vi "DLIbufferedRead.vi"(9 "timeout(ms)":i32, 10 "Ch.":i32, 11 "URL":string) -> (0 "error out":errorcluster, 1 "state(1or0)":i16, 2 "body":string, 3 "headers":string)   [LabVIEW 2016]
uses:
  DLIbufferState.ctl
  ADAM Client/Sub VIs/ADAM Controls/Remember_value_mode.ctl
  <vilib>/httpClient/LabVIEWHTTPClient.lvlib
panel:
  out "allChs":u32 format="%08b"
  out "age(s)":dbl
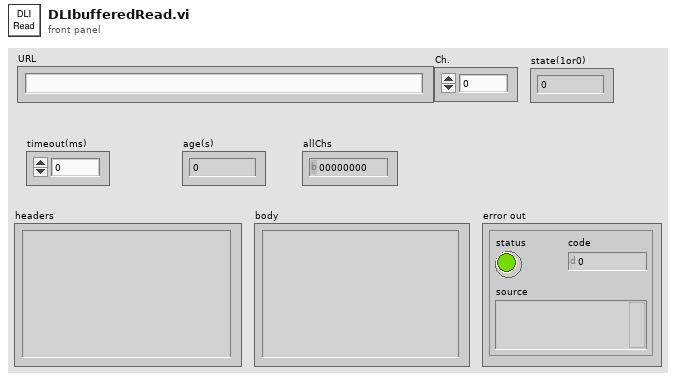
[diagram p1: front panel]
types:
  T1 = typedef "DLIbufferState.ctl" = enum16{"CheckStoredAge", "UseStoredValue", "Read", "Store"}
  T2 = typedef "Remember_value_mode.ctl" = enum16{"Read only", "Read and Write"}
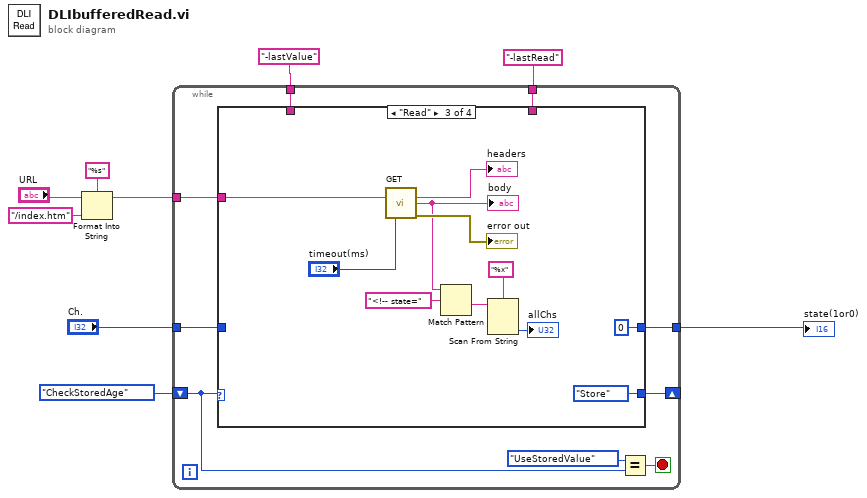
[diagram p0: block diagram]
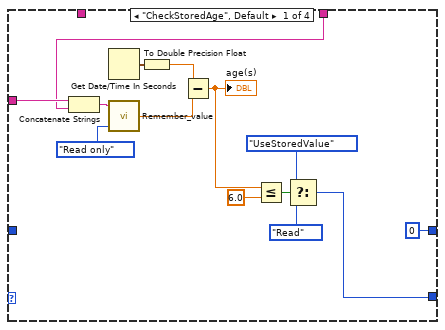
[diagram p2: hidden frame]
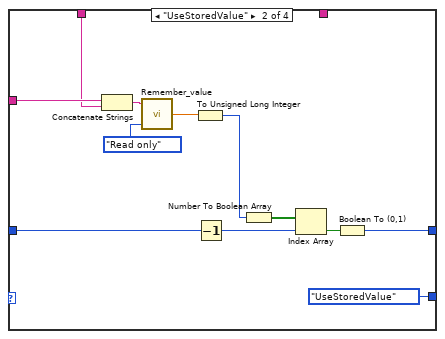
[diagram p3: hidden frame]
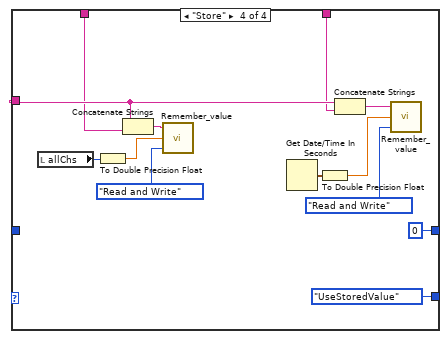
[diagram p4: hidden frame]
diagram:
  n1 = Format Into String(format string="%s", initial string="URL", "/index.htm" ("input 1")) -> (resulting string=w5:string)  [unwired: 1 in, 1 out]
  n2 = while {
    shift-right: [w15] -> _
    shift-left: DLIbufferState."CheckStoredAge" -> [w10]
    tunnel: w5 -> [w18]
    tunnel: "Ch." -> [w17]
    tunnel: [w16] -> w3
    tunnel: "-lastRead" ("string") -> [w14]
    tunnel: "-lastValue" ("string") -> [w13]
    stop <- w12 stop-if-true
    n3 = case shown="\"Read\"" w10 {
      tunnel: w18 -> [w29 w42 w48 w62]
      tunnel: w17 -> [_ w36 _ _]
      tunnel: [i16 0 w35 i16 0 i16 0] -> w16
      tunnel: [w22 DLIbufferState."UseStoredValue" DLIbufferState."Store" DLIbufferState."UseStoredValue"] -> w15
      tunnel: w14 -> [w19 _ _ w59]
      tunnel: w13 -> [_ w34 _ w58]
      frame "CheckStoredAge", Default {
        n4 = Concatenate Strings(w29, w19) -> (w30:string)
        n5 = Get Date/Time In Seconds() -> (seconds since 1Jan1904=w32:timestamp)
        n6 = call "Remember_value.vi"("Mode"=Remember_value_mode."Read only", "Ch name"=w30) -> ("Output Value"=w27:dbl)  [unwired: 1 in]
        n7 = To Double Precision Float(number=w32) -> (double precision float=w28:dbl)
        n8 = Subtract(x=w28, y=w27) -> (x-y=w26:dbl)
        "age(s)" <- w26
        n9 = Less Or Equal?(x=w26, y=6.0) -> (x <= y?=w24:bool)
        n10 = Select(t=DLIbufferState."UseStoredValue", s=w24, f=DLIbufferState."Read") -> (s? t:f=w22:T1)
      }
      frame "UseStoredValue" {
        n11 = Concatenate Strings(w42, w34) -> (w44:string)
        n12 = call "Remember_value.vi"("Mode"=Remember_value_mode."Read only", "Ch name"=w44) -> ("Output Value"=w38:dbl)  [unwired: 1 in]
        n13 = To Unsigned Long Integer(number=w38) -> (unsigned 32bit integer=w37:u32)
        n14 = Decrement(x=w36) -> (x-1=w40:i32)
        n15 = Number To Boolean Array(number=w37) -> (Boolean array=w39:bool[])
        n16 = Index Array(array=w39, index=w40) -> (element=w41:bool)
        n17 = Boolean To (0,1)(Boolean=w41) -> (0, 1=w35:i16)
      }
      frame "Read" {
        n18 = call <vilib>:"GET.vi"("url"=w48, "timeout (10000)"="timeout(ms)") -> ("headers"=→"headers":string, "body"=w50:string, "error out"=→"error out":errorcluster)  [unwired: 10 in, 1 out]
        "body" <- w50
        n19 = Match Pattern(string=w50, regular expression="<!-- state=") -> (after substring=w54:string)  [unwired: 1 in, 3 out]
        n20 = Scan From String(format string="%x", input string=w54) -> (output 1=→"allChs":u32)  [unwired: 3 in, 3 out]
      }
      frame "Store" {
        n21 = local read "allChs"() -> (w61:u32)
        n22 = To Double Precision Float(number=w61) -> (double precision float=w60:dbl)
        n23 = Concatenate Strings(w62, w58) -> (w68:string)
        n24 = call "Remember_value.vi"("Mode"=Remember_value_mode."Read and Write", "Input Value"=w60, "Ch name"=w68) -> ()  [unwired: 1 out]
        n25 = Get Date/Time In Seconds() -> (seconds since 1Jan1904=w65:timestamp)
        n26 = To Double Precision Float(number=w65) -> (double precision float=w66:dbl)
        n27 = Concatenate Strings(w62, w59) -> (w63:string)
        n28 = call "Remember_value.vi"("Mode"=Remember_value_mode."Read and Write", "Input Value"=w66, "Ch name"=w63) -> ()  [unwired: 1 out]
      }
    }
    n29 = Equal?(x=DLIbufferState."UseStoredValue", y=w10) -> (x = y?=w12:bool)
  }
  "state(1or0)" <- w3
